vi "__Driver_interaction_Test.vi"() -> ()   [LabVIEW 2014, in "Driver_interaction.lvlib"]
uses:
  Driver_interaction.lvlib
  _Driver_interaction/Controls/Driver_interaction_instrument_type.ctl
  _Driver_interaction/Controls/Interface_type.ctl
  Toolbox/Controls/Group_output.ctl
  Toolbox/Controls/Group_selector.ctl
  _Driver_interaction/_Driver_interaction.lvclass
  Toolbox/Toolbox.lvclass
panel:
  out "Devices_Addressed":i32
  in  "Addressing":bool
  in  "Group_output":T1
  in  "value_to_write":dbl
  in  "Command write":bool
  in  "command_write":string
  in  "Dimming":bool
  in  "Channel_output":dbl[](array[numeric])
  in  "Command read":bool
  out "responses":string[](array[string])
  in  "command_read":string
  out "devices_found":i32
  in  "Interface_type":T3="DALI"
  in  "Instrument_type":T4="Toolbox"
  out "error out":errorcluster
  in  "error in (no error)":errorcluster
  # "DMX"
  # "DALI"
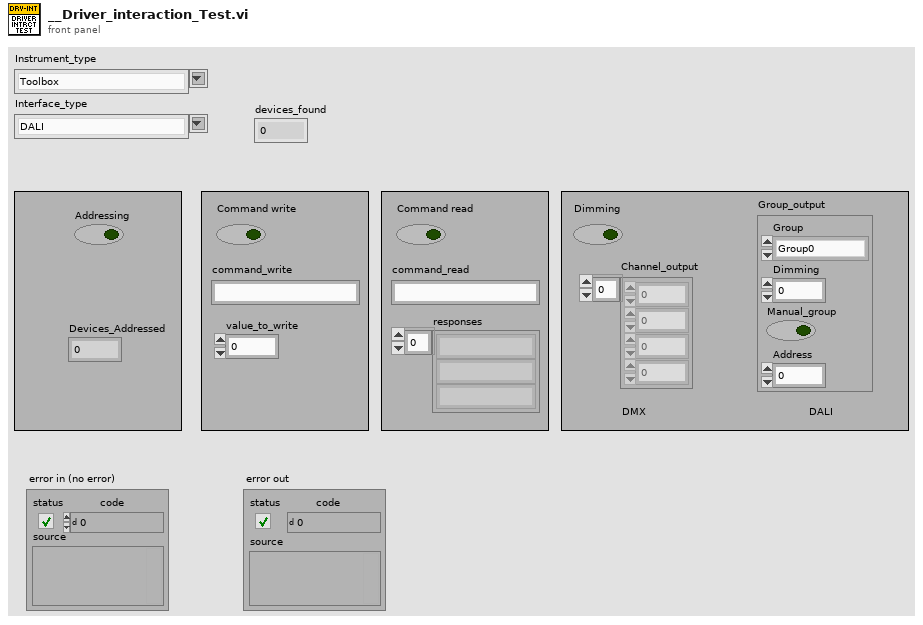
[diagram p1: front panel]
types:
  T1 = typedef "Driver_interaction.lvlib/Toolbox.lvclass/Group_output.ctl" = cluster{"Group":T2, "Dimming":i32, "Manual_group":bool, "Address":i32}
  T2 = typedef "Driver_interaction.lvlib/Toolbox.lvclass/Group_selector.ctl" = enum16{"Group0", "Group1", "Group2", "Group3", "Group4", "Group5", "Group6", "Group7", "Group8", "Group9", "Group10", "Group11", "Group12", "Group13", "Group14", "Group15", "All Groups"}
  T3 = typedef "Driver_interaction.lvlib/_Driver_interaction.lvclass/Interface_type.ctl" = string
  T4 = typedef "Driver_interaction.lvlib/_Driver_interaction.lvclass/Driver_interaction_instrument_type.ctl" = string
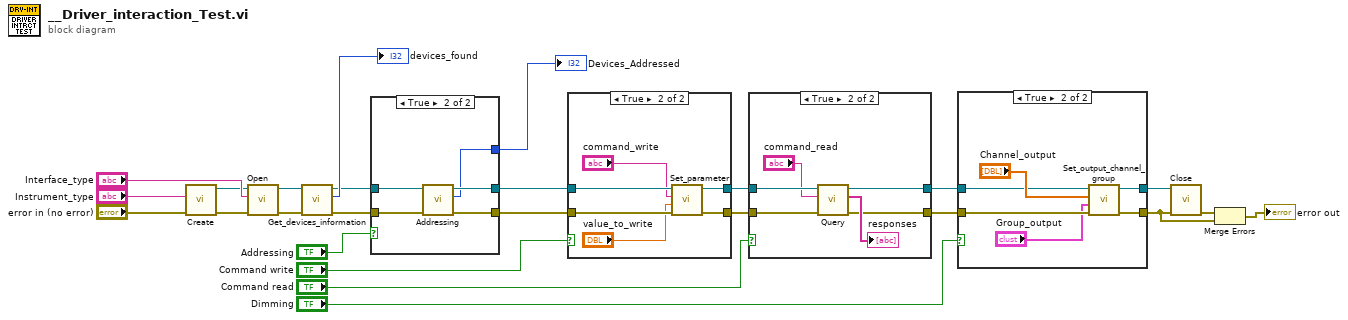
[diagram p0: block diagram]
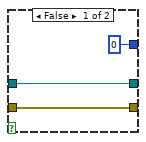
[diagram p2: hidden frame]
diagram:
  n1 = call "Create.vi"("error in (no error)"="error in (no error)", "Instrument_type"="Instrument_type") -> ("error out"=w21:errorcluster, "_Driver_interaction out"=w22:refnum<class "_Driver_interaction.lvclass">)  [unwired: 8 in]
  n2 = call-dynamic "Open.vi"("error in (no error)"=w21, "Interface_type"="Interface_type", "_Driver_interaction in"=w22) -> ("error out"=w20:errorcluster, "_Driver_interaction out"=w19:refnum<class "_Driver_interaction.lvclass">)  [unwired: 7 in]
  n3 = call-dynamic "Get_devices_information.vi"("error in (no error)"=w20, "_Driver_interaction in"=w19) -> ("error out"=w5:errorcluster, "devices_found"=→"devices_found":i32, "_Driver_interaction out"=w6:refnum<class "_Driver_interaction.lvclass">)  [unwired: 7 in]
  n4 = case shown="True" "Addressing" {
    tunnel: w6 -> [w28 w33]
    tunnel: w5 -> [w27 w32]
    tunnel: [w27 w31] -> w4
    tunnel: [w28 w30] -> w3
    tunnel: [0 ("Dispositivos") w29] -> w1
    frame False {
    }
    frame True {
      n5 = call-dynamic "Addressing.vi"("error in (no error)"=w32, "_Driver_interaction in"=w33) -> ("error out"=w31:errorcluster, "Devices_Addresed"=w29:i32, "_Driver_interaction out"=w30:refnum<class "_Driver_interaction.lvclass">)  [unwired: 7 in]
    }
  }
  "Devices_Addressed" <- w1
  n6 = case shown="True" "Command write" {
    tunnel: [w35 w41] -> w9
    tunnel: w4 -> [w34 w40]
    tunnel: w3 -> [w35 w39]
    tunnel: [w34 w38] -> w8
    frame False {
    }
    frame True {
      n7 = call-dynamic "Set_parameter.vi"("error in (no error)"=w40, "value"="value_to_write", "parameter"="command_write", "_Driver_interaction in"=w39) -> ("error out"=w38:errorcluster, "_Driver_interaction out"=w41:refnum<class "_Driver_interaction.lvclass">)  [unwired: 6 in]
    }
  }
  n8 = case shown="True" "Command read" {
    tunnel: [w43 w48] -> w14
    tunnel: w8 -> [w42 w47]
    tunnel: w9 -> [w43 w46]
    tunnel: [w42 w45] -> w13
    frame False {
    }
    frame True {
      n9 = call-dynamic "Query.vi"("error in (no error)"=w47, "command"="command_read", "_Driver_interaction in"=w46) -> ("error out"=w45:errorcluster, "responses"=→"responses":string[], "_Driver_interaction out"=w48:refnum<class "_Driver_interaction.lvclass">)  [unwired: 6 in]
    }
  }
  n10 = case shown="True" "Dimming" {
    tunnel: w14 -> [w51 w56]
    tunnel: w13 -> [w50 w55]
    tunnel: [w50 w54] -> w12
    tunnel: [w51 w53] -> w11
    frame False {
    }
    frame True {
      n11 = call-dynamic "Set_output_channel_group.vi"("error in (no error)"=w55, "Group_output"="Group_output", "Channel_output"="Channel_output", "_Driver_interaction in"=w56) -> ("error out"=w54:errorcluster, "_Driver_interaction out"=w53:refnum<class "_Driver_interaction.lvclass">)  [unwired: 6 in]
    }
  }
  n12 = call-dynamic "Close.vi"("error in (no error)"=w12, "_Driver_interaction in"=w11) -> ("error out"=w17:errorcluster)  [unwired: 8 in, 1 out]
  n13 = Merge Errors(w17, w12) -> (→"error out":errorcluster)
